vi "Convert Readback Register Info for Bridge.vi"(5 "Reg_Address_to_Read":T1={"First Reg Address"=31, "Num of Reg to Read"=31} {"Num of Reg to Read" min=1; "First Reg Address" format="%.0x"}) -> (2 "number":u32 format="%.0x")   [LabVIEW 2013]
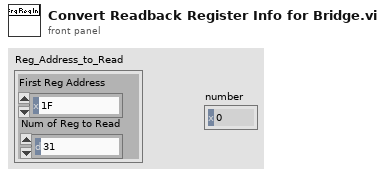
[diagram p1: front panel]
types:
  T1 = cluster{"First Reg Address":u8, "Num of Reg to Read":u8}
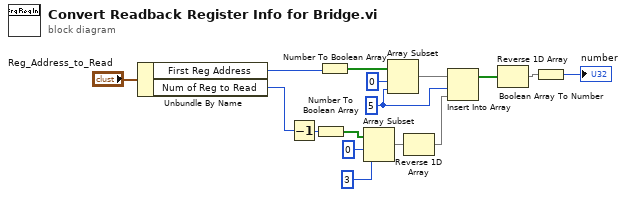
[diagram p0: block diagram]
diagram:
  w7 = 5 ("length")
  n1 = Unbundle By Name("Reg_Address_to_Read") -> ("First Reg Address"=w15:u8, "Num of Reg to Read"=w2:u8)
  n2 = Decrement(x=w2) -> (x-1=w1:u8)
  n3 = Number To Boolean Array(number=w1) -> (Boolean array=w9:bool[])
  n4 = Number To Boolean Array(number=w15) -> (Boolean array=w14:bool[])
  n5 = Array Subset(array=w9, index=0, length=3) -> (w6:bool[])
  n6 = Array Subset(array=w14, index=0, length=w7) -> (w8:bool[])
  n7 = Reverse 1D Array(array=w6) -> (reversed array=w3:bool[])
  n8 = Insert Into Array(array=w8, index=w7, new element=w3) -> (w5:bool[])
  n9 = Reverse 1D Array(array=w5) -> (reversed array=w4:bool[])
  n10 = Boolean Array To Number(Boolean array=w4) -> (number=→"number":u32)
